vi "convert palette names into relative paths.vi"(11 "palettes":T1(array[cluster])) -> (3 "nested palettes":T1(array[cluster]))   [LabVIEW 2020]
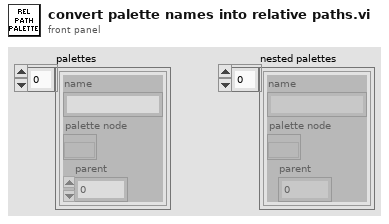
[diagram p1: front panel]
types:
  T1 = cluster{"name":string, "palette node":refnum<k20>, "parent":i32}[]
  T2 = cluster{"name":string, "palette node":refnum<k20>, "parent":i32}
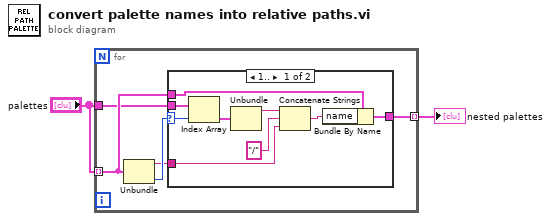
[diagram p0: block diagram]
diagram:
  n1 = for {
    tunnel: "palettes" -> [w6] mode=indexing
    tunnel: "palettes" -> [w3]
    tunnel: [w5] -> w2 mode=indexing
    n2 = Unbundle(w6) -> ("name"=w4:string, "parent"=w7:i32)  [unwired: 1 out]
    n3 = case shown="1.." w7 {
      selector: w7 -> [w13 _]
      tunnel: w6 -> [w16 w17]
      tunnel: [w15 w17] -> w5
      tunnel: w4 -> [w11 _]
      tunnel: w3 -> [w14 _]
      frame 1.. {
        n4 = Index Array(array=w14, index=w13) -> (element=w12:T2)
        n5 = Unbundle(w12) -> ("name"=w8:string)  [unwired: 2 out]
        n6 = Concatenate Strings(w8, "/" ("string"), w11) -> (w10:string)
        n7 = Bundle By Name(cluster=w16, "name"=w10) -> (w15:T2)
      }
      frame ..0 {
      }
    }
  }
  "nested palettes" <- w2
